vi "To String (Array).vi"(6 "pretty print? (T)":bool=TRUE, 7 "enable LabVIEW extensions? (T)":bool=TRUE, 8 "error in (no error)":errorcluster, 10 "indent":i32, 11 "JSON Value in":variant) -> (0 "error out":errorcluster, 3 "String":string)   [LabVIEW 2017, in "Advanced Variant Tools.lvlib"]
doc: "Flattens the given JSON data to a string."
uses:
  Advanced Variant Tools.lvlib
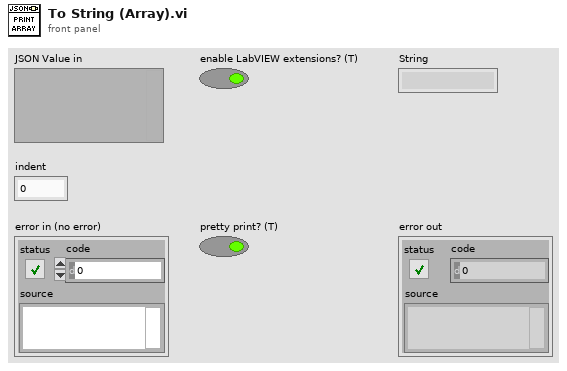
[diagram p1: front panel]
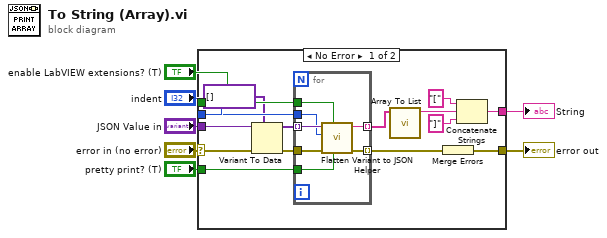
[diagram p0: block diagram]
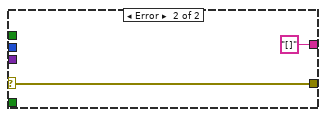
[diagram p2: hidden frame]
diagram:
  n1 = case shown="No Error" "error in (no error)" {
    selector: "error in (no error)" -> [w12 w31]
    tunnel: "JSON Value in" -> [w14 _]
    tunnel: [w20 w31] -> w5
    tunnel: [w19 "[]"] -> w4
    tunnel: "enable LabVIEW extensions? (T)" -> [w15 _]
    tunnel: "pretty print? (T)" -> [w10 _]
    tunnel: "indent" -> [w9 _]
    frame No Error {
      n2 = Variant To Data(error in=w12, type=variant[] [], Variant=w14) -> (data=w13:variant[], error out=w11:errorcluster)
      n3 = for {
        tunnel: [w29] -> w22 mode=indexing
        tunnel: w11 -> [w28]
        tunnel: [w27] -> w21 mode=indexing
        tunnel: w15 -> [w26]
        tunnel: w13 -> [w25] mode=indexing
        tunnel: w10 -> [w24]
        tunnel: w9 -> [w23]
        n4 = call "Flatten Variant to JSON Helper.vi"("pretty print? (T)"=w24, "enable LabVIEW extensions? (T)"=w26, "error in (no error)"=w28, "indent"=w23, "JSON Value in"=w25) -> ("error out"=w27:errorcluster, "String"=w29:string)  [unwired: 5 in]
      }
      n5 = call "Array To List.vi"("Array"=w22) -> ("String"=w18:string)  [unwired: 10 in]
      n6 = Merge Errors(w21) -> (w20:errorcluster)
      n7 = Concatenate Strings("[" ("string"), w18, "]" ("string")) -> (w19:string)
    }
    frame Error {
    }
  }
  "String" <- w4
  "error out" <- w5
